vi "single_animal_subimage_pixel_ranges.vi"(9 "Input \nparameters":T2={"Frame rate (ms)"=2000, "Worm strain"="N2", "# Images"=0, "State"=enum."Image acquisition", "Time elapsed"=0.0, "Max_num_runs"=100000, "#TTL"=0, "Time of start TTL"=100000, "ImSub Value"=0, "Time of last TTL"=0, "# Animals per column"=2, "# Animals per row"=2, "# AdjacentTTL"=0, "Sleep deprivation status"="", "Sleep Detection"=FALSE, "# Sleep detections"=0, "Time of first sleep detection"=0, "Time max # adjacent TTL"=0, "Image t-1"=[], "Image t"=[]} {"# Animals per row" items=["1"=1, "2"=2, "3"=3, "4"=4]; "# Animals per column" items=["1"=1, "2"=2, "3"=3, "4"=4]}, 11 "Action":T4) -> (1 "Single animal\nsubimage pixel\nranges":T3)   [LabVIEW 2011]
uses:
  Action Items.ctl
  state.ctl
panel:
  out "?":i32
  out "?":i32
  in  "Single animal\nsubimage pixels":T3
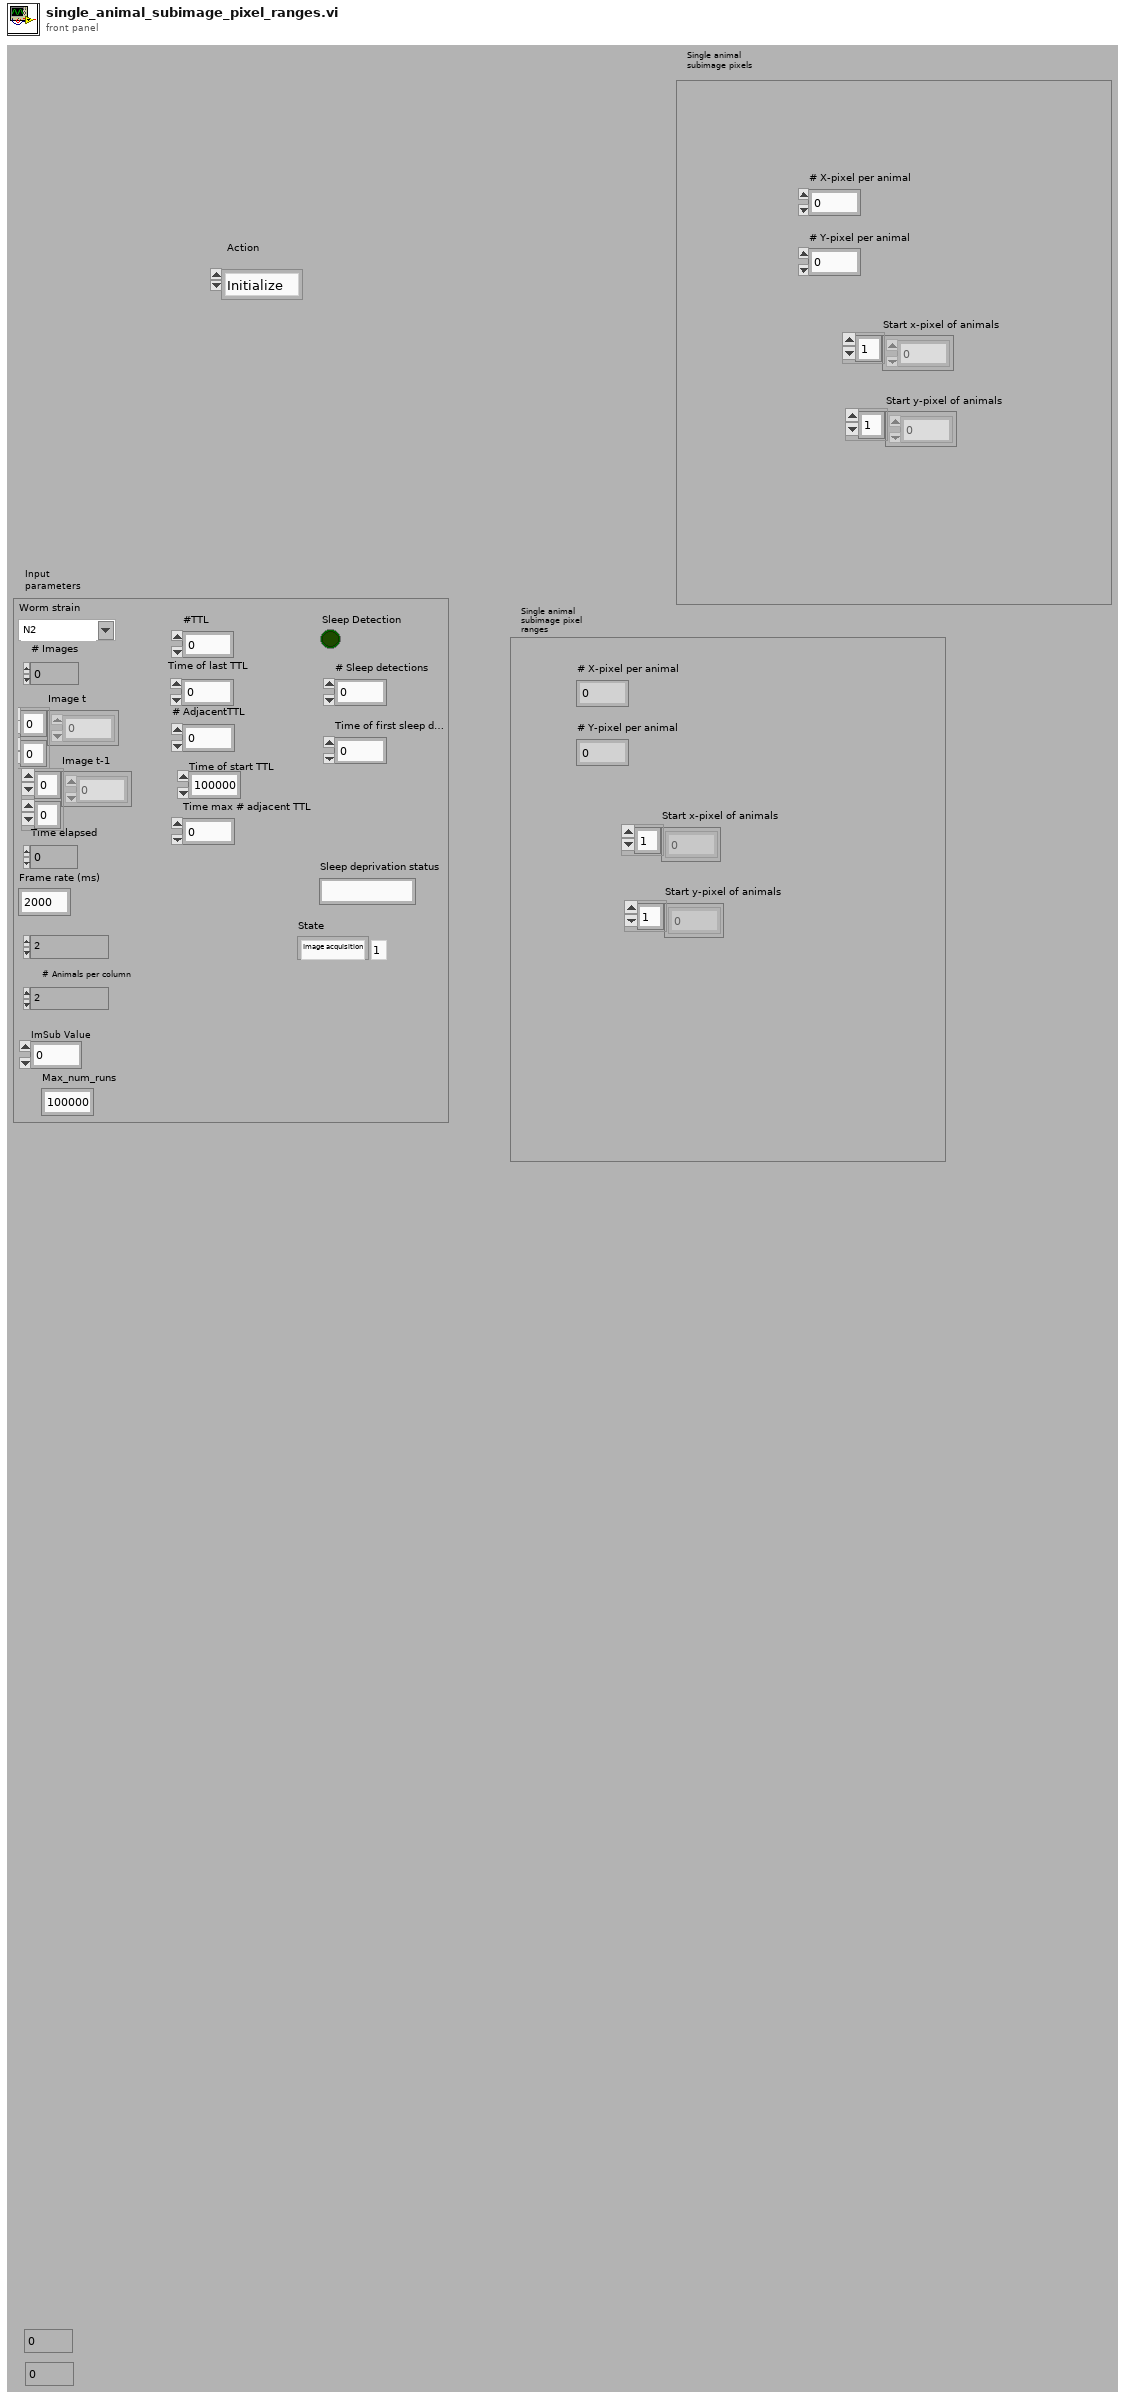
[diagram p1: front panel]
types:
  T1 = typedef "state.ctl" = enum16{"Initialize measurement", "Image acquisition", "Image processing", "Sleep detection", "Control TTL protocol ", "Sleep deprivation", "Update image & exit condition", "Wait "}
  T2 = cluster{"Frame rate (ms)":u32, "Worm strain":string, "# Images":i32, "State":T1, "Time elapsed":dbl, "Max_num_runs":i32, "#TTL":i32, "Time of start TTL":i32, "ImSub Value":i32, "Time of last TTL":i32, "# Animals per column":u32, "# Animals per row":u32, "# AdjacentTTL":i32, "Sleep deprivation status":string, "Sleep Detection":bool, "# Sleep detections":i32, "Time of first sleep detection":i32, "Time max # adjacent TTL":i32, "Image t-1":i32[][], "Image t":i32[][]}
  T3 = cluster{"# X-pixel per animal":i32, "# Y-pixel per animal":i32, "Start x-pixel of animals":i32[], "Start y-pixel of animals":i32[]}
  T4 = typedef "Action Items.ctl" = enum16{"Initialize", "Get"}
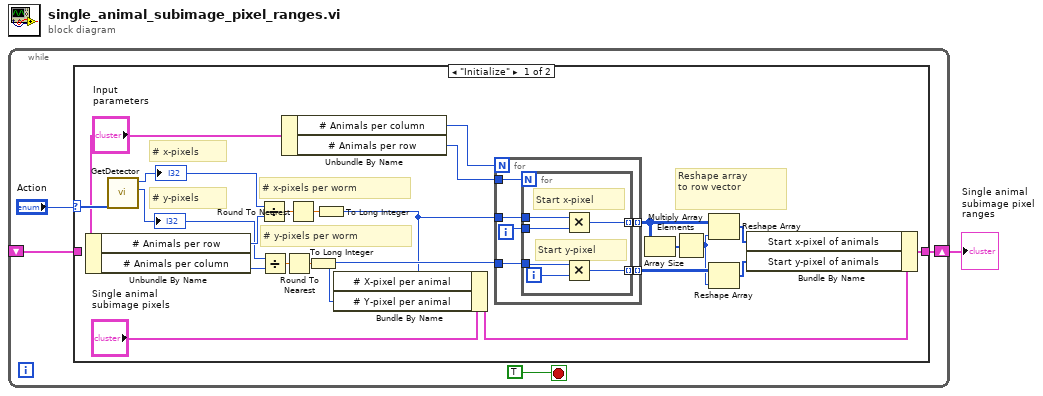
[diagram p0: block diagram]
diagram:
  n1 = while {
    shift-right: [w2] -> w1
    shift-left: _ -> [w3]
    stop <- TRUE ("stop") stop-if-true
    n2 = case shown="\"Initialize\"" "Action" {
      tunnel: w3 -> [_ w40]
      tunnel: [w16 w40] -> w2
      frame "Initialize" {
        # "Reshape array \nto row vector"
        # "# y-pixels"
        # "# x-pixels"
        # "# x-pixels per worm"
        # "# y-pixels per worm"
        n3 = Unbundle By Name("Input \nparameters") -> ("# Animals per row"=w24:u32, "# Animals per column"=w25:u32)
        n4 = call <userlib>:"GetDetector.vi"() -> ("ypixels"=w7:i32, "xpixels"=w6:i32)  [unwired: 4 in, 2 out]
        "?" <- w6
        "?" <- w7
        n5 = Divide(x=w6, y=w24) -> (x/y=w26:dbl)
        n6 = Divide(x=w7, y=w25) -> (x/y=w27:dbl)
        n7 = Unbundle By Name("Input \nparameters") -> ("# Animals per column"=w14:u32, "# Animals per row"=w13:u32)
        n8 = Round To Nearest(number=w27) -> (nearest integer value=w18:dbl)
        n9 = Round To Nearest(number=w26) -> (nearest integer value=w19:dbl)
        n10 = To Long Integer(number=w18) -> (32bit integer=w9:i32)
        n11 = To Long Integer(number=w19) -> (32bit integer=w8:i32)
        n12 = Bundle By Name(cluster="Single animal\nsubimage pixels", "# X-pixel per animal"=w8, "# Y-pixel per animal"=w9) -> (w20:T3)
        n13 = for {
          N: w14 -> [_]
          tunnel: w13 -> [w33]
          tunnel: w8 -> [w31]
          tunnel: w9 -> [w30]
          tunnel: [w29] -> w12 mode=indexing
          tunnel: [w28] -> w23 mode=indexing
          i -> [w32]
          n14 = for {
            N: w33 -> [_]
            tunnel: w32 -> [w34]
            tunnel: w31 -> [w35]
            tunnel: w30 -> [w38]
            tunnel: [w37] -> w29 mode=indexing
            tunnel: [w36] -> w28 mode=indexing
            i -> [w39]
            # "Start y-pixel"
            # "Start x-pixel"
            n15 = Multiply(x=w35, y=w34) -> (x*y=w37:i32)
            n16 = Multiply(x=w38, y=w39) -> (x*y=w36:i32)
          }
        }
        n17 = Array Size(array=w12) -> (size(s)=w11:i32[])
        n18 = Multiply Array Elements(1:w11) -> (0:w10:i32)
        n19 = Reshape Array(w12, w10) -> (w21:i32[])
        n20 = Reshape Array(w23, w10) -> (w22:i32[])
        n21 = Bundle By Name(cluster=w20, "Start x-pixel of animals"=w21, "Start y-pixel of animals"=w22) -> (w16:T3)
      }
      frame "Get" {
      }
    }
  }
  "Single animal\nsubimage pixel\nranges" <- w1
